vi "Point to Distance on Board.vi"(2 "Size of square":i16, 3 "scaled value":i16) -> (0 "end pixel":i16, 1 "start pixel":i16)   [LabVIEW 2023]
doc: "Given a point in the 11x7 grid, translate that into pixels in the board's coordinates for a square that will cover 2 grid squares."
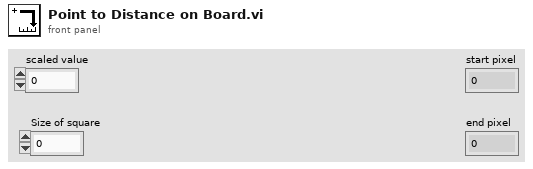
[diagram p1: front panel]
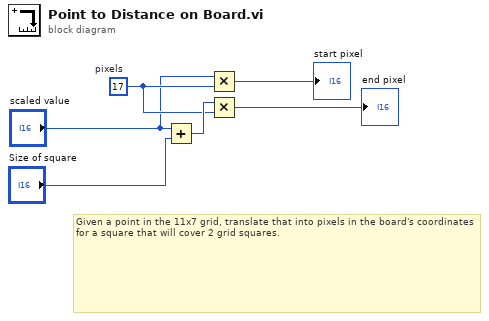
[diagram p0: block diagram]
diagram:
  w3 = i16 17  # pixels
  # "Given a point in the 11x7 grid, translate that into pixels in the board's coordinates for a square that will cover 2 grid squares."
  n1 = Add(x="scaled value", y="Size of square") -> (x+y=w4:i16)
  n2 = Multiply(x="scaled value", y=w3) -> (x*y=→"start pixel":i16)
  n3 = Multiply(x=w4, y=w3) -> (x*y=→"end pixel":i16)
